vi "Convert Thermistor Reading (scaler).vi"(0 "Voltage":sgl=1.25 format="%0.4f", 1 "Type of Excitation":u16(ring) items=["Voltage Reference", "Current Reference"], 2 "Voltage Reference":sgl=2.5 format="%0.2f", 3 "R1":sgl=5000.0 format="%0.2f", 4 "Excitation Current":sgl=0.0001 format="%0.2e", 7 "Temperature Units (C)":u16(ring) items=["Celsius", "Fahrenheit", "Kelvin", "Rankine"]) -> (5 "Temperature":sgl=25.0 format="%0.2f")   [LabVIEW 2013]
doc: "Converts a thermistor voltage into temperature."
panel:
  # "Vo"
  # "Common Applications:  \n{Rt is the thermistor located in the isothermal terminal block. a, b and c are specific for the particular thermistor.}\n\nVoltage Source:\nFor our calculations, R1 is 5kOhms, Rt (Resistance for the thermistor) at 25 degrees Celsius is 5 kOhms, and Vref = 2.5V.\nThe calculated temperature (T) is in Kelvin and is converted to Celsius.\n\nCurrent Source:\nThe DAQPad MIO-16XE-50 card, for example, provides a constant current source at 100 micro Amps, which can be used to excite the thermistor.\n\nIn this case It = 100 micro Amps and Rt at 25 degrees Celsius is 5kOhms with Vo = 0.5V.\n\nNI 435x (Temperature) Devices:\nThe built-in CJC sensor on the 435x accessories is a thermistor.\nHowever, the ConvertThermocouple Reading VI assumes that a thermistor CJC sensor uses voltage excitation.\nThe thermistor on the accessory is read in Ohms mode for greater accuracy, and by playing a trick on the Convert Thermistor Reading VI, we can get an IC Sensor equivalent voltage so that the Convert Thermocouple Reading VI can convert the reading to a temperature."
  # "V ref"
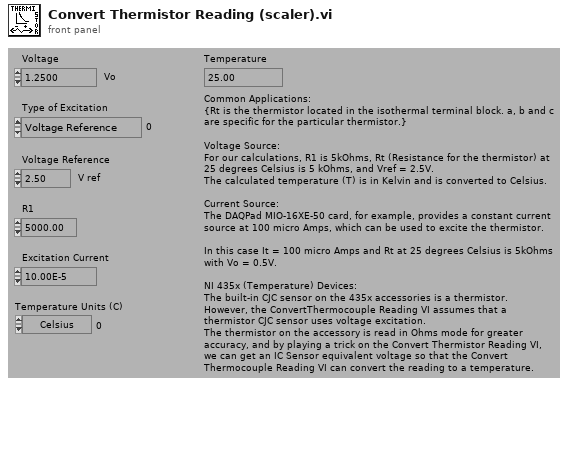
[diagram p1: front panel]
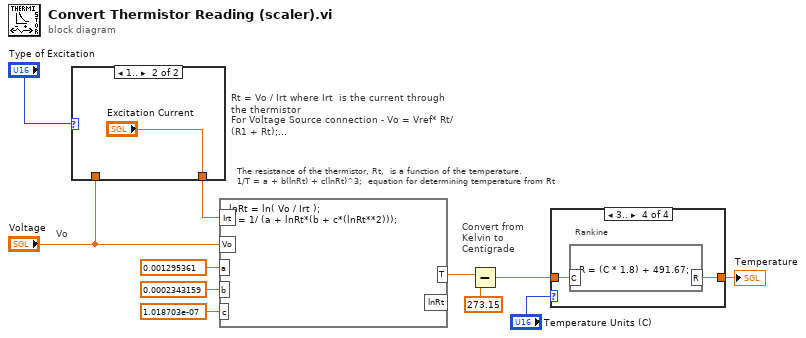
[diagram p0: block diagram]
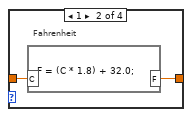
[diagram p3: hidden frame]
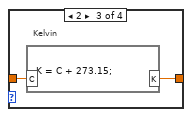
[diagram p4: hidden frame]
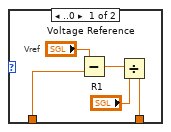
[diagram p5: hidden frame]
diagram:
  # "The resistance of the thermistor, Rt,  is a function of the temperature.\n1/T = a + b(lnRt) + c(lnRt)^3;  equation for determining temperature from Rt"
  # "Vo"
  # "Convert from \nKelvin to \nCentigrade"
  n1 = case "Rt = Vo / Irt where Irt  is the current through the thermistor\nFor Voltage Source connection - Vo = Vref* Rt/ (R1 + Rt); \n     or Rt = R1 ( Vo / (Vref - Vo))\n     Irt = R1 / (Vref - Vo)\nFor Current Source connection - Vo = Iex * Rt\n     or Rt = Vo / Iex\n     Irt = Iex" shown="1.." "Type of Excitation" {
    tunnel: "Voltage" -> [w15 _]
    tunnel: [w13 "Excitation Current"] -> w6
    frame ..0 {
      # "Vref"
      n2 = Subtract(x="Voltage Reference", y=w15) -> (x-y=w16:sgl)
      n3 = Divide(x=w16, y="R1") -> (x/y=w13:sgl)
    }
    frame 1.. {
    }
  }
  n4 = formula code="lnRt = ln( Vo / Irt );\nT = 1/ (a + lnRt*(b + c*(lnRt**2)));"("Vo"="Voltage", "a"=0.001295361, "b"=0.0002343159, "c"=1.018703e-07, "Irt"=w6) -> ("T"=w8:dbl)  [unwired: 1 out]
  n5 = Subtract(x=w8, y=273.15) -> (x-y=w2:dbl)
  n6 = case shown="3.." "Temperature Units (C)" {
    tunnel: w2 -> [w18 w20 w22 w24]
    tunnel: [w18 w19 w21 w23] -> w1
    frame ..0 {
      # "Celsius"
    }
    frame 1 {
      # "Fahrenheit"
      n7 = formula code="F = (C * 1.8) + 32.0;"("C"=w20) -> ("F"=w19:dbl)
    }
    frame 2 {
      # "Kelvin"
      n8 = formula code="K = C + 273.15;"("C"=w22) -> ("K"=w21:dbl)
    }
    frame 3.. {
      # "Rankine"
      n9 = formula code="R = (C * 1.8) + 491.67;"("C"=w24) -> ("R"=w23:dbl)
    }
  }
  "Temperature" <- w1
